vi "convert_voltage_to_turn.vi"(4 "bypass_valve_v0":dbl format="%#_13g", 5 "coef_bv":dbl=0.967 format="%#_13g", 6 "run_valve_v0":dbl format="%#_13g", 7 "coef_rv":dbl=0.967 format="%#_13g", 8 "status_in":bool, 10 "bypass_valve_voltage":dbl, 11 "run_valve_voltage":dbl) -> (0 "status_out":bool, 2 "bypass_valve_turn":dbl, 3 "run_valve_turn":dbl)   [LabVIEW 2019]
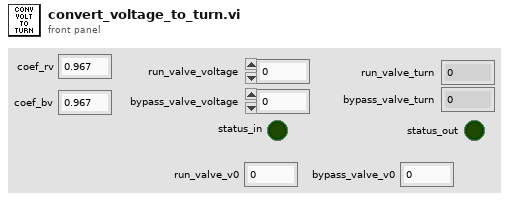
[diagram p1: front panel]
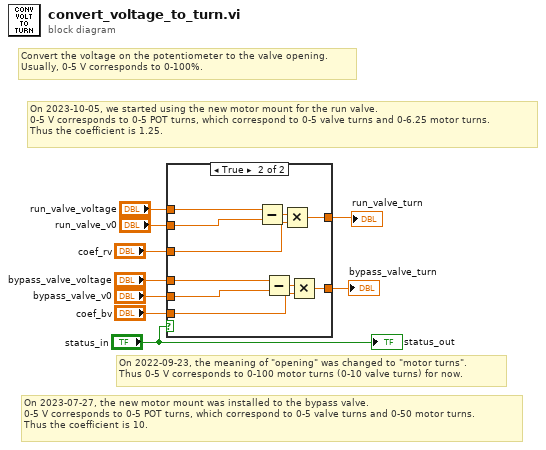
[diagram p0: block diagram]
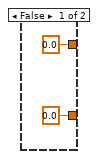
[diagram p2: hidden frame]
diagram:
  # "On 2023-10-05, we started using the new motor mount for the run valve.\n0-5 V corresponds to 0-5 POT turns, which correspond to 0-5 valve turns and 0-6.25 motor turns.\nThus the coefficient is 1.25."
  # "On 2023-07-27, the new motor mount was installed to the bypass valve.\n0-5 V corresponds to 0-5 POT turns, which correspond to 0-5 valve turns and 0-50 motor turns.\nThus the coefficient is 10."
  # "On 2022-09-23, the meaning of \"opening\" was changed to \"motor turns\".\nThus 0-5 V corresponds to 0-100 motor turns (0-10 valve turns) for now."
  # "Convert the voltage on the potentiometer to the valve opening.\nUsually, 0-5 V corresponds to 0-100%."
  n1 = case shown="True" "status_in" {
    tunnel: [0.0 w19] -> w9
    tunnel: [0.0 w18] -> w8
    tunnel: "run_valve_voltage" -> [_ w17]
    tunnel: "bypass_valve_voltage" -> [_ w15]
    tunnel: "run_valve_v0" -> [_ w16]
    tunnel: "bypass_valve_v0" -> [_ w14]
    tunnel: "coef_rv" -> [_ w13]
    tunnel: "coef_bv" -> [_ w12]
    frame False {
    }
    frame True {
      n2 = Subtract(x=w17, y=w16) -> (x-y=w21:dbl)
      n3 = Subtract(x=w15, y=w14) -> (x-y=w20:dbl)
      n4 = Multiply(x=w21, y=w13) -> (x*y=w19:dbl)
      n5 = Multiply(x=w20, y=w12) -> (x*y=w18:dbl)
    }
  }
  "run_valve_turn" <- w9
  "bypass_valve_turn" <- w8
  "status_out" <- "status_in"
